vi "gyroscope mecanum thing.vi"() -> ()   [LabVIEW 2019]
panel:
  in  "Direction":dbl
  in  "Target Position":dbl
  in  "stop":bool
  out "backRight":dbl
  out "backLeft":dbl
  out "frontRight":dbl
  out "frontLeft":dbl
  in  "gyroscope position":dbl
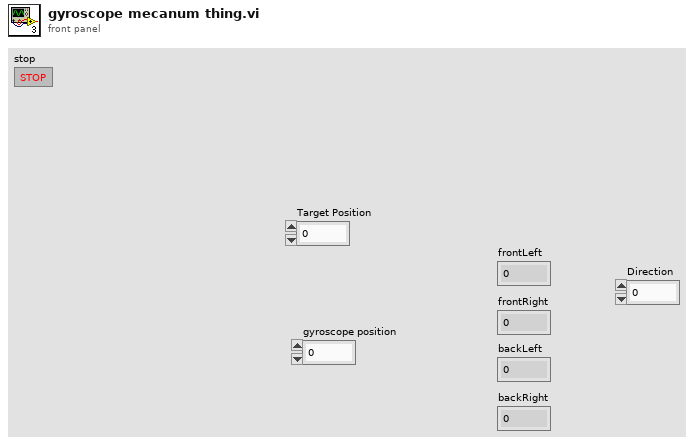
[diagram p1: front panel]
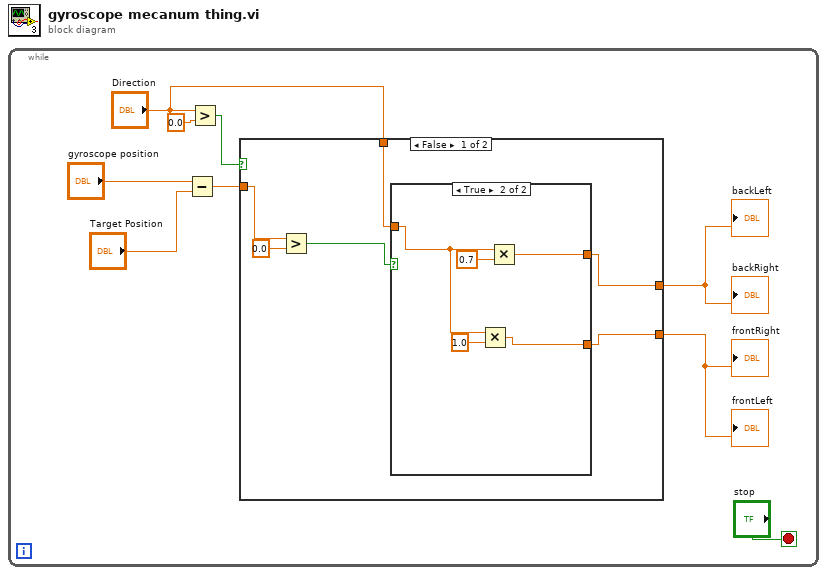
[diagram p0: block diagram]
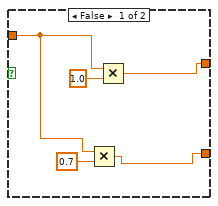
[diagram p2: hidden frame]
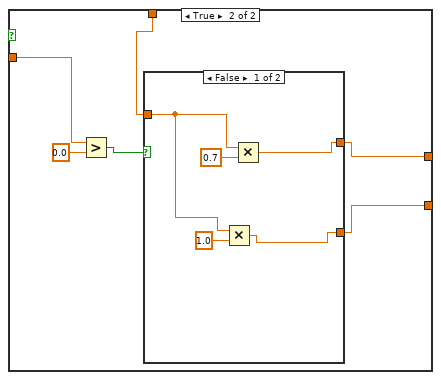
[diagram p3: hidden frame]
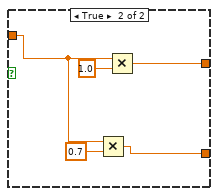
[diagram p4: hidden frame]
diagram:
  n1 = while {
    stop <- "stop" stop-if-true
    n2 = Subtract(x="gyroscope position", y="Target Position") -> (x-y=w4:dbl)
    n3 = Greater?(x="Direction", y=0.0) -> (0:w5:bool)
    n4 = case shown="False" w5 {
      tunnel: w4 -> [w15 w29]
      tunnel: [w11 w27] -> w3
      tunnel: [w10 w26] -> w2
      tunnel: "Direction" -> [w12 w31]
      frame False {
        n5 = Greater?(x=w15, y=0.0) -> (0:w13:bool)
        n6 = case shown="True" w13 {
          tunnel: w12 -> [w16 w25]
          tunnel: [w18 w22] -> w11
          tunnel: [w17 w21] -> w10
          frame False {
            n7 = Multiply(x=w16, y=0.7) -> (x*y=w17:dbl)
            n8 = Multiply(x=w16, y=1.0) -> (x*y=w18:dbl)
          }
          frame True {
            n9 = Multiply(x=w25, y=1.0) -> (x*y=w21:dbl)
            n10 = Multiply(x=w25, y=0.7) -> (x*y=w22:dbl)
          }
        }
      }
      frame True {
        n11 = Greater?(x=w29, y=0.0) -> (0:w28:bool)
        n12 = case shown="False" w28 {
          tunnel: w31 -> [w32 w41]
          tunnel: [w34 w38] -> w27
          tunnel: [w33 w37] -> w26
          frame False {
            n13 = Multiply(x=w32, y=1.0) -> (x*y=w33:dbl)
            n14 = Multiply(x=w32, y=0.7) -> (x*y=w34:dbl)
          }
          frame True {
            n15 = Multiply(x=w41, y=0.7) -> (x*y=w37:dbl)
            n16 = Multiply(x=w41, y=1.0) -> (x*y=w38:dbl)
          }
        }
      }
    }
    "frontLeft" <- w2
    "frontRight" <- w2
    "backLeft" <- w3
    "backRight" <- w3
  }
